vi "labview_nanonisKernel.vi"(3 "Error in (no error)":errorcluster, 4 "Input":string, 5 "Application ref in":refnum<vi>) -> (0 "Error out":errorcluster, 2 "Output":string)   [LabVIEW 2019]
uses:
  <userlib>/Nanonis Prog Interface/Scan/Grid/GridPatternGet.vi
  <userlib>/Nanonis Prog Interface/Nanonis Prog Interface.lvlib
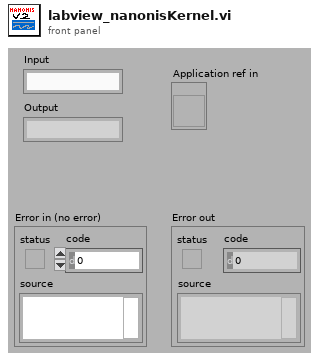
[diagram p1: front panel]
types:
  T1 = enum16{"no change", "home absolute", "home relative"}
  T2 = enum8{"Group 1", "Group 2", "Group 3", "Group 4", "Group 5", "Group 6"}
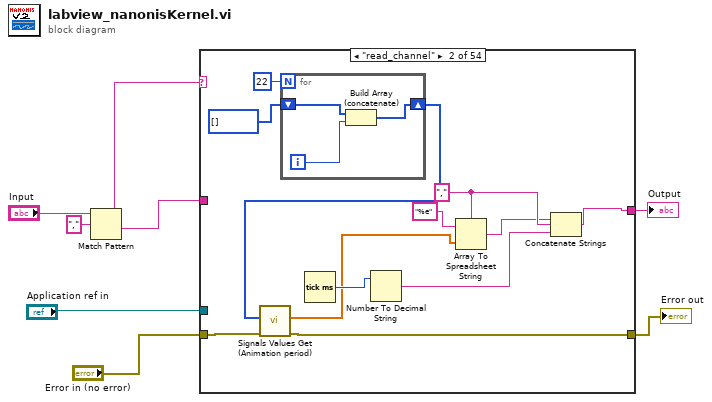
[diagram p0: block diagram]
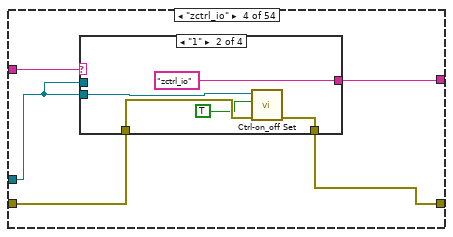
[diagram p4: hidden frame]
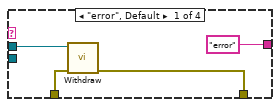
[diagram p5: hidden frame]
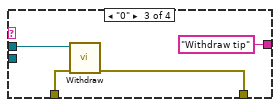
[diagram p6: hidden frame]
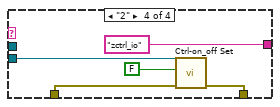
[diagram p7: hidden frame]
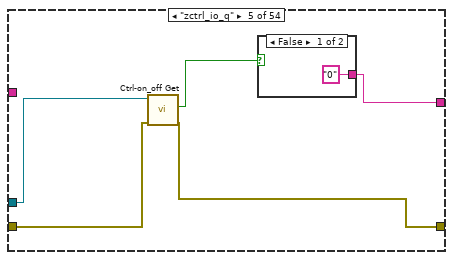
[diagram p8: hidden frame]
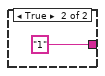
[diagram p9: hidden frame]
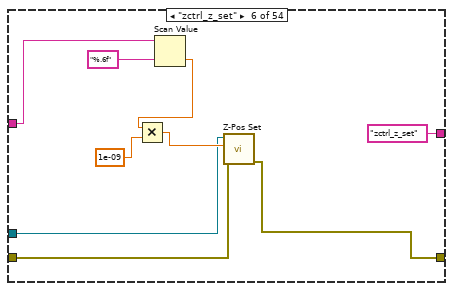
[diagram p10: hidden frame]
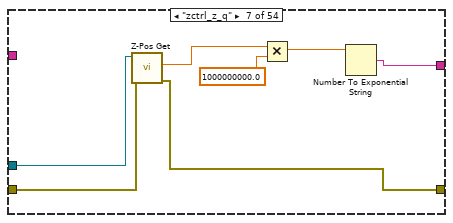
[diagram p11: hidden frame]
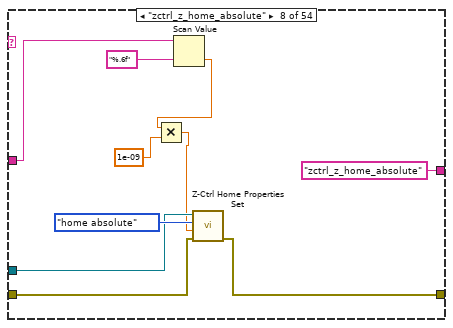
[diagram p12: hidden frame]
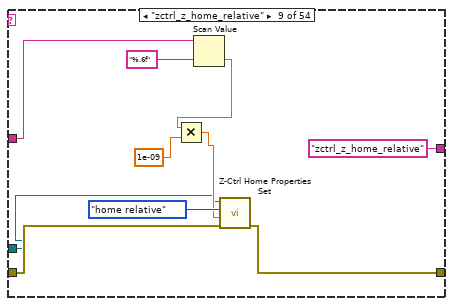
[diagram p13: hidden frame]
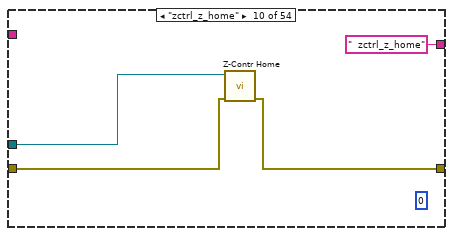
[diagram p14: hidden frame]
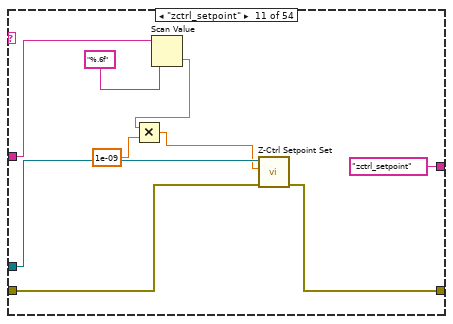
[diagram p15: hidden frame]
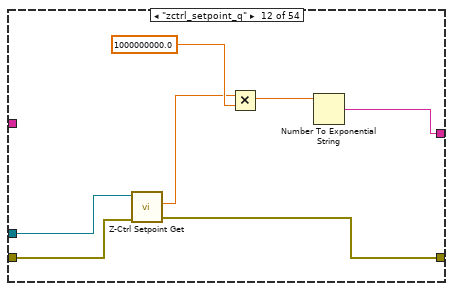
[diagram p16: hidden frame]
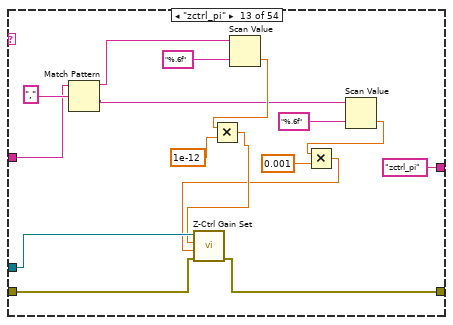
[diagram p17: hidden frame]
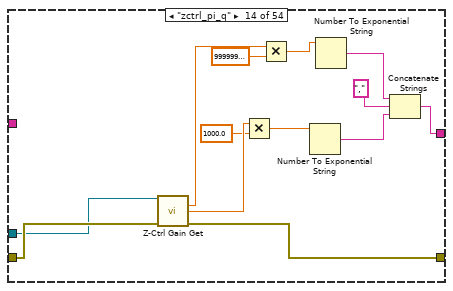
[diagram p18: hidden frame]
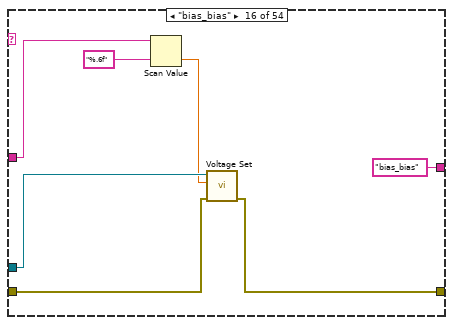
[diagram p20: hidden frame]
diagram:
  n1 = Match Pattern(string="Input", regular expression=",") -> (before substring=w5:string, after substring=w4:string)  [unwired: 1 in, 2 out]
  n2 = case shown="\"read_channel\"" w5 {
    tunnel: [w10 w12 w27 w31 w52 "zctrl_z_set" ("Input") w68 "zctrl_z_home_absolute" ("Input") "zctrl_z_home_relative" ("Input") "  zctrl_z_home" ("Input") "zctrl_setpoint" ("Input") w111 "zctrl_pi" ("Input") w130 w144 "bias_bias" ("Input") w153 "bias_pulse" ("Input") w176 w197 "bias_spec_sweep" ("Input") w216 "  bias_spec_channel" ("Input") w234 w241 w244 "walker_setting" ("Input") w264 "walker_walk" ("Input") " walker_uni_walk " ("Input") "walker_stop" ("regular expression") w344 "move_move" ("regular expression") "move_stop" ("regular expression") w370 "  move_speed" ("regular expression") w389 w397 w399 w401 w406 "lockin_setting" ("regular expression") w435 "lockin_channel" ("regular expression") w460 w479 w495 w507 w515 w530 w538 "1" ("regular expression") w552 w566] -> w8
    tunnel: w4 -> [w10 _ w27 w32 _ w65 _ w74 w84 _ w98 _ w121 _ w144 w145 _ w164 w178 _ w204 _ w230 w234 _ w244 w248 _ w270 w318 _ w344 w349 _ _ w384 _ w397 w399 w401 w402 w428 _ w451 _ w471 w496 _ w526 _ _ _ _ _]
    tunnel: "Error in (no error)" -> [w9 w22 w26 w30 w54 w60 w72 w81 w91 w97 w106 w109 w128 w142 w143 w151 w156 w171 w180 w195 w212 w221 w229 w233 w239 w243 w255 w263 w268 w325 w343 w345 w362 w366 w378 w388 w395 w396 w398 w400 w405 w434 w445 w457 w466 w486 w494 w506 _ w536 w541 w550 w556 w572]
    tunnel: "Application ref in" -> [_ _ _ w29 w55 w61 w73 w79 w85 w94 w105 w110 w127 w140 _ w148 w155 w170 w177 w194 w210 w213 w227 _ w238 _ w256 w261 w269 w326 w342 _ w361 w365 w376 w387 w393 _ _ _ w403 w432 w444 w456 w465 w487 w493 w504 w518 w537 w542 w548 w555 w573]
    tunnel: [w9 w21 w26 w28 w51 w58 w67 w80 w90 w96 w104 w108 w126 w141 w143 w150 w154 w169 w179 w196 w211 w220 w228 w233 w240 w243 w254 w262 w267 w324 w341 w345 w360 w364 w377 w380 w394 w396 w398 w400 w404 w433 w443 w455 w464 w485 w490 w505 w517 w535 w539 w549 w554 w571] -> w2
    frame "test", Default {
    }
    frame "read_channel" {
      w16 = "," ("delimiter (Tab)")
      n3 = for {
        N: 22 -> [_]
        shift-right: [w24] -> w18
        shift-left: i32[] [] -> [w25]
        i -> [w23]
        n4 = Build Array (concatenate)(w25, w23) -> (w24:i32[])
      }
      n5 = call <userlib>:"Signals Values Get (Animation period).vi"("error in (no error)"=w22, "Signals indexes (0-23)"=w18) -> ("error out"=w21:errorcluster, "Signals Values"=w11:sgl[])  [unwired: 6 in, 1 out]
      n6 = Tick Count (ms)() -> (millisecond timer value=w15:u32)
      n7 = Number To Decimal String(number=w15) -> (decimal integer string=w13:string)  [unwired: 1 in]
      n8 = Array To Spreadsheet String(delimiter (Tab)=w16, array=w11, 3:"%e" ("format string")) -> (spreadsheet string=w14:string)
      n9 = Concatenate Strings(w14, w16, w13) -> (w12:string)
    }
    frame "###z controller###" {
    }
    frame "zctrl_io" {
      n10 = case shown="\"1\"" w32 {
        tunnel: ["error" ("regular expression") "zctrl_io" ("regular expression") "Withdraw tip" ("regular expression") "zctrl_io" ("regular expression")] -> w31
        tunnel: w29 -> [w34 _ w45 _]
        tunnel: w30 -> [w35 w40 w44 w46]
        tunnel: w29 -> [_ w38 _ w48]
        tunnel: [w33 w37 w42 w49] -> w28
        frame "error", Default {
          n11 = call <userlib>:"Withdraw.vi"("Error in (no error)"=w35, "Application ref in"=w34) -> ("Error out"=w33:errorcluster)  [unwired: 8 in, 1 out]
        }
        frame "1" {
          n12 = call <userlib>:"Ctrl-on_off Set.vi"("error in (no error)"=w40, "Z Controller ON/OFF"=TRUE ("Lockin ON/OFF"), "Application ref in"=w38) -> ("error out"=w37:errorcluster)  [unwired: 7 in, 1 out]
        }
        frame "0" {
          n13 = call <userlib>:"Withdraw.vi"("Error in (no error)"=w44, "Application ref in"=w45) -> ("Error out"=w42:errorcluster)  [unwired: 8 in, 1 out]
        }
        frame "2" {
          n14 = call <userlib>:"Ctrl-on_off Set.vi"("error in (no error)"=w46, "Z Controller ON/OFF"=FALSE ("Lockin ON/OFF"), "Application ref in"=w48) -> ("error out"=w49:errorcluster)  [unwired: 7 in, 1 out]
        }
      }
    }
    frame "zctrl_io_q" {
      n15 = call <userlib>:"Ctrl-on_off Get.vi"("error in (no error)"=w54, "Application ref in"=w55) -> ("error out"=w51:errorcluster, "Z-Controller on/off status"=w53:bool)  [unwired: 7 in, 1 out]
      n16 = case shown="False" w53 {
        tunnel: ["0" "1"] -> w52
        frame False {
        }
        frame True {
        }
      }
    }
    frame "zctrl_z_set" {
      n17 = Scan Value(string=w65, format string="%.6f") -> (value=w63:dbl)  [unwired: 1 in, 1 out]
      n18 = Multiply(x=w63, y=1e-09) -> (x*y=w62:dbl)
      n19 = call <userlib>:"Z-Pos Set.vi"("error in (no error)"=w60, "Z position (m)"=w62, "Application ref in"=w61) -> ("error out"=w58:errorcluster)  [unwired: 7 in, 1 out]
    }
    frame "zctrl_z_q" {
      n20 = call <userlib>:"Z-Pos Get.vi"("error in (no error)"=w72, "Application ref in"=w73) -> ("error out"=w67:errorcluster, "Z position (m)"=w70:sgl)  [unwired: 7 in, 1 out]
      n21 = Multiply(x=w70, y=1000000000.0) -> (x*y=w69:dbl)
      n22 = Number To Exponential String(number=w69) -> (E-format string=w68:string)  [unwired: 3 in]
    }
    frame "zctrl_z_home_absolute" {
      n23 = Scan Value(string=w74, format string="%.6f") -> (value=w76:dbl)  [unwired: 1 in, 1 out]
      n24 = Multiply(x=w76, y=1e-09) -> (x*y=w75:dbl)
      n25 = call <userlib>:"Z-Ctrl Home Properties Set.vi"("error in (no error)"=w81, "Home position (m) (NaN=no change)"=w75, "Absolute/Relative Switch (no change=Default)"=T1."home absolute", "Application ref in"=w79) -> ("error out"=w80:errorcluster)  [unwired: 5 in, 1 out]
    }
    frame "zctrl_z_home_relative" {
      n26 = Scan Value(string=w84, format string="%.6f") -> (value=w87:dbl)  [unwired: 1 in, 1 out]
      n27 = Multiply(x=w87, y=1e-09) -> (x*y=w86:dbl)
      n28 = call <userlib>:"Z-Ctrl Home Properties Set.vi"("error in (no error)"=w91, "Home position (m) (NaN=no change)"=w86, "Absolute/Relative Switch (no change=Default)"=T1."home relative", "Application ref in"=w85) -> ("error out"=w90:errorcluster)  [unwired: 5 in, 1 out]
    }
    frame "zctrl_z_home" {
      (unwired) 0
      n29 = call <userlib>:"Z-Contr Home.vi"("Error in (no error)"=w97, "Application ref in"=w94) -> ("Error out"=w96:errorcluster)  [unwired: 8 in, 1 out]
    }
    frame "zctrl_setpoint" {
      n30 = Scan Value(string=w98, format string="%.6f") -> (value=w101:dbl)  [unwired: 1 in, 1 out]
      n31 = Multiply(x=w101, y=1e-09) -> (x*y=w100:dbl)
      n32 = call <userlib>:"Z-Ctrl Setpoint Set.vi"("error in (no error)"=w106, "Z Controller setpoint"=w100, "Application ref in"=w105) -> ("error out"=w104:errorcluster)  [unwired: 7 in, 1 out]
    }
    frame "zctrl_setpoint_q" {
      n33 = call <userlib>:"Z-Ctrl Setpoint Get.vi"("error in (no error)"=w109, "Application ref in"=w110) -> ("error out"=w108:errorcluster, "Z Controller setpoint"=w107:sgl)  [unwired: 6 in, 1 out]
      n34 = Multiply(x=w107, y=1000000000.0) -> (x*y=w112:dbl)
      n35 = Number To Exponential String(number=w112) -> (E-format string=w111:string)  [unwired: 3 in]
    }
    frame "zctrl_pi" {
      n36 = Match Pattern(string=w121, regular expression=",") -> (before substring=w120:string, after substring=w117:string)  [unwired: 1 in, 2 out]
      n37 = Scan Value(string=w120, format string="%.6f") -> (value=w123:dbl)  [unwired: 1 in, 1 out]
      n38 = Multiply(x=w123, y=1e-12) -> (x*y=w119:dbl)
      n39 = Scan Value(string=w117, format string="%.6f") -> (value=w116:dbl)  [unwired: 1 in, 1 out]
      n40 = Multiply(x=w116, y=0.001) -> (x*y=w115:dbl)
      n41 = call <userlib>:"Z-Ctrl Gain Set.vi"("error in (no error)"=w128, "Time constant (s)"=w115, "P-gain"=w119, "Application ref in"=w127) -> ("error out"=w126:errorcluster)  [unwired: 5 in, 1 out]
    }
    frame "zctrl_pi_q" {
      n42 = call <userlib>:"Z-Ctrl Gain Get.vi"("Application ref in"=w140, "error in (no error)"=w142) -> ("P-gain"=w137:sgl, "Time constant (s)"=w136:sgl, "error out"=w141:errorcluster)  [unwired: 9 in, 2 out]
      n43 = Multiply(x=w136, y=sgl 1000.0) -> (x*y=w138:sgl)
      n44 = Multiply(x=w137, y=sgl 1000000000000.0) -> (x*y=w139:sgl)
      n45 = Number To Exponential String(number=w138) -> (E-format string=w131:string)  [unwired: 3 in]
      n46 = Number To Exponential String(number=w139) -> (E-format string=w132:string)  [unwired: 3 in]
      n47 = Concatenate Strings(w132, "," ("string"), w131) -> (w130:string)
    }
    frame "###Bias/Bias Spectrum###" {
    }
    frame "bias_bias" {
      n48 = Scan Value(string=w145, format string="%.6f") -> (value=w147:dbl)  [unwired: 1 in, 1 out]
      n49 = call <userlib>:"Voltage Set.vi"("Error in (no error)"=w151, "Bias (V)"=w147, "Application ref in"=w148) -> ("Error out"=w150:errorcluster)  [unwired: 7 in, 1 out]
    }
    frame "bias_bias_q" {
      n50 = call <userlib>:"Voltage Get.vi"("error in (no error)"=w156, "Application ref in"=w155) -> ("error out"=w154:errorcluster, "Bias (V)"=w152:sgl)  [unwired: 7 in, 1 out]
      n51 = Number To Exponential String(number=w152) -> (E-format string=w153:string)  [unwired: 3 in]
    }
    frame "bias_pulse" {
      w161 = "," ("regular expression")
      n52 = Match Pattern(string=w164, regular expression=w161) -> (before substring=w166:string, after substring=w159:string)  [unwired: 1 in, 2 out]
      n53 = Match Pattern(string=w159, regular expression=w161) -> (before substring=w160:string, after substring=w158:string)  [unwired: 1 in, 2 out]
      n54 = Scan Value(string=w166, format string="%.6f") -> (value=w163:dbl)  [unwired: 1 in, 1 out]
      n55 = case shown="\"0\"" w158 {
        tunnel: [enum16{"no change", "hold", "don't hold"}."no change" ("Z-Controller (no change)") enum16{"no change", "hold", "don't hold"}."hold" ("Z-Controller (no change)") enum16{"no change", "hold", "don't hold"}."don't hold" ("Z-Controller (no change)")] -> w157
        frame Default {
        }
        frame "1" {
        }
        frame "0" {
        }
      }
      n56 = Scan Value(string=w160, format string="%.6f") -> (value=w162:dbl)  [unwired: 1 in, 1 out]
      n57 = call <userlib>:"Bias Pulse.vi"("Application ref in"=w170, "Pulse bias (V) (1)"=w163, "Pulse width (s) (100m)"=w162, "Z-Controller (no change)"=w157, "Error in (no error)"=w171, "Pulse abs/rel (no change)"=enum16{"no change", "relative", "absolute"}."absolute") -> ("Error out"=w169:errorcluster)  [unwired: 8 in, 1 out]
    }
    frame "bias_spec_io" {
      n58 = case shown="\"1\"" w178 {
        tunnel: ["Error!" ("regular expression") w185 "STS stop" ("regular expression")] -> w176
        tunnel: w180 -> [w181 w189 w192]
        tunnel: w177 -> [_ w190 _]
        tunnel: [w181 w188 w191] -> w179
        frame "error", Default {
        }
        frame "1" {
          n59 = call <userlib>:"BiasSpectroscopy Start.vi"("Application ref in"=w190, "Get data (F)"=TRUE, "Error in (no error)"=w189) -> ("Data"=w184:sgl[][], "Error out"=w188:errorcluster)  [unwired: 8 in, 3 out]
          n60 = Array To Spreadsheet String(delimiter (Tab)=",", array=w184, 3:"%e" ("format string")) -> (spreadsheet string=w185:string)
        }
        frame "0" {
          n61 = call <userlib>:"BiasSpectroscopy Stop.vi"("Error in (no error)"=w192) -> ("Error out"=w191:errorcluster)  [unwired: 13 in, 1 out]
        }
      }
    }
    frame "bias_spec_q" {
      n62 = call <userlib>:"BiasSpectroscopy Status Get.vi"("Error in (no error)"=w195, "Application ref in"=w194) -> ("Error out"=w196:errorcluster, "Running?"=w198:bool)  [unwired: 5 in, 1 out]
      n63 = case shown="True" w198 {
        tunnel: ["0" "1"] -> w197
        frame False {
        }
        frame True {
        }
      }
    }
    frame "bias_spec_sweep" {
      n64 = Match Pattern(string=w204, regular expression=",") -> (before substring=w207:string, after substring=w205:string)  [unwired: 1 in, 2 out]
      n65 = Scan Value(string=w207, format string="%.6f") -> (value=w203:dbl)  [unwired: 1 in, 1 out]
      n66 = Scan Value(string=w205, format string="%.6f") -> (value=w202:dbl)  [unwired: 1 in, 1 out]
      n67 = call <userlib>:"BiasSpectroscopy SetLimits.vi"("Error in (no error)"=w212, "End value (V)"=w202, "Start value (V)"=w203, "Application ref in"=w210) -> ("Error out"=w211:errorcluster)  [unwired: 4 in, 1 out]
    }
    frame "bias_spec_sweep_q" {
      n68 = call <userlib>:"BiasSpectroscopy GetLimits.vi"("Error in (no error)"=w221, "Application ref in"=w213) -> ("Error out"=w220:errorcluster, "End value (V)"=w215:sgl, "Start value (V)"=w214:sgl)  [unwired: 4 in, 1 out]
      n69 = Number To Exponential String(number=w215) -> (E-format string=w217:string)  [unwired: 3 in]
      n70 = Number To Exponential String(number=w214) -> (E-format string=w218:string)  [unwired: 3 in]
      n71 = Concatenate Strings(w218, "," ("string"), w217) -> (w216:string)
    }
    frame "bias_spec_channel" {
      n72 = Spreadsheet String To Array(delimiter (Tab)=",", format string="", spreadsheet string=w230) -> (array=w225:dbl[][])  [unwired: 1 in]
      n73 = Array Size(array=w225) -> (size(s)=w226:i32[])
      n74 = Array Max & Min(array=w226) -> (max value=w224:i32)  [unwired: 3 out]
      n75 = Reshape Array(w225, w224) -> (w223:dbl[])
      n76 = call <userlib>:"BiasSpectroscopy Channels Set.vi"("Error in (no error)"=w229, "Channels"=w223, "Application ref in"=w227) -> ("Error out"=w228:errorcluster)  [unwired: 7 in, 1 out]
    }
    frame "###Current###" {
    }
    frame "current" {
      n77 = call <userlib>:"Current Get.vi"("Error in (no error)"=w239, "Application ref in"=w238) -> ("Error out"=w240:errorcluster, "Current (A)"=w237:sgl)  [unwired: 5 in, 1 out]
      n78 = Multiply(x=sgl 1000000000.0, y=w237) -> (x*y=w236:sgl)
      n79 = Format Value(format string="%e", value (0)=w236) -> (output string=w241:string)  [unwired: 1 in]
    }
    frame "###Walker###" {
    }
    frame "walker_setting" {
      n80 = Match Pattern(string=w248, regular expression=",") -> (before substring=w251:string, after substring=w249:string)  [unwired: 1 in, 2 out]
      n81 = Scan Value(string=w251, format string="%.6f") -> (value=w247:dbl)  [unwired: 1 in, 1 out]
      n82 = Scan Value(string=w249, format string="%.6f") -> (value=w246:dbl)  [unwired: 1 in, 1 out]
      n83 = call <userlib>:"Motor Frequency Amplitude Set.vi"("Error in (no error)"=w255, "Amplitude (V) (NaN=no change)"=w247, "Frequency (Hz) (NaN=no change)"=w246, "Application ref in"=w256) -> ("Error out"=w254:errorcluster)  [unwired: 6 in, 1 out]
    }
    frame "walker_setting_q" {
      n84 = call <userlib>:"Motor Frequency Amplitude Get.vi"("Error in (no error)"=w263, "Application ref in"=w261) -> ("Error out"=w262:errorcluster, "Amplitude (V)"=w260:sgl, "Frequency (Hz)"=w258:sgl)  [unwired: 6 in, 1 out]
      n85 = Number To Decimal String(number=w258) -> (decimal integer string=w257:string)  [unwired: 1 in]
      n86 = Number To Decimal String(number=w260) -> (decimal integer string=w259:string)  [unwired: 1 in]
      n87 = Concatenate Strings(w259, "," ("string"), w257) -> (w264:string)
    }
    frame "walker_walk" {
      n88 = Match Pattern(string=w270, regular expression=",") -> (before substring=w275:string, after substring=w273:string)  [unwired: 1 in, 2 out]
      n89 = Scan Value(string=w275, format string="%d") -> (value=w271:dbl)  [unwired: 1 in, 1 out]
      n90 = Scan Value(string=w273, format string="%d") -> (value=w272:dbl)  [unwired: 1 in, 1 out]
      n91 = case shown="2" w271 {
        tunnel: w269 -> [_ w284 w290 w296 w302 w308 w310]
        tunnel: w268 -> [w278 w283 w289 w295 w301 w307 w313]
        tunnel: [w278 w282 w288 w294 w300 w306 w312] -> w267
        tunnel: w272 -> [_ w280 w286 w292 w298 w304 w311]
        frame 0, Default {
        }
        frame 1 {
          n92 = call <userlib>:"Motor Start Move.vi"("Group"=T2."Group 4", "Error in (no error)"=w283, "Number of steps"=w280, "Direction"=enum16{"X +", "X -", "Y +", "Y -", "Z +", "Z -"}."X +", "Application ref in"=w284) -> ("Error out"=w282:errorcluster)  [unwired: 4 in, 1 out]
        }
        frame 2 {
          n93 = call <userlib>:"Motor Start Move.vi"("Group"=T2."Group 4", "Error in (no error)"=w289, "Number of steps"=w286, "Direction"=enum16{"X +", "X -", "Y +", "Y -", "Z +", "Z -"}."X -", "Application ref in"=w290) -> ("Error out"=w288:errorcluster)  [unwired: 4 in, 1 out]
        }
        frame 3 {
          n94 = call <userlib>:"Motor Start Move.vi"("Group"=T2."Group 4", "Error in (no error)"=w295, "Number of steps"=w292, "Direction"=enum16{"X +", "X -", "Y +", "Y -", "Z +", "Z -"}."Y +", "Application ref in"=w296) -> ("Error out"=w294:errorcluster)  [unwired: 4 in, 1 out]
        }
        frame 4 {
          n95 = call <userlib>:"Motor Start Move.vi"("Group"=T2."Group 4", "Error in (no error)"=w301, "Number of steps"=w298, "Direction"=enum16{"X +", "X -", "Y +", "Y -", "Z +", "Z -"}."Y -", "Application ref in"=w302) -> ("Error out"=w300:errorcluster)  [unwired: 4 in, 1 out]
        }
        frame 5 {
          n96 = call <userlib>:"Motor Start Move.vi"("Group"=T2."Group 4", "Error in (no error)"=w307, "Number of steps"=w304, "Direction"=enum16{"X +", "X -", "Y +", "Y -", "Z +", "Z -"}."Z +", "Application ref in"=w308) -> ("Error out"=w306:errorcluster)  [unwired: 4 in, 1 out]
        }
        frame 6 {
          n97 = call <userlib>:"Motor Start Move.vi"("Group"=T2."Group 4", "Error in (no error)"=w313, "Number of steps"=w311, "Direction"=enum16{"X +", "X -", "Y +", "Y -", "Z +", "Z -"}."Z -", "Application ref in"=w310) -> ("Error out"=w312:errorcluster)  [unwired: 4 in, 1 out]
        }
      }
    }
    frame "walker_uni_walk" {
      n98 = Match Pattern(string=w318, regular expression=",") -> (before substring=w321:string, after substring=w319:string)  [unwired: 1 in, 2 out]
      n99 = Scan Value(string=w321, format string="%d") -> (value=w316:dbl)  [unwired: 1 in, 1 out]
      n100 = Scan Value(string=w319, format string="%d") -> (value=w317:dbl)  [unwired: 1 in, 1 out]
      n101 = case shown="0, Default" w316 {
        tunnel: w326 -> [_ w333 w335]
        tunnel: w325 -> [w327 w332 w338]
        tunnel: [w327 w331 w337] -> w324
        tunnel: w317 -> [_ w329 w336]
        frame 0, Default {
        }
        frame 5 {
          n102 = call <userlib>:"Motor Start Move.vi"("Group"=T2."Group 5", "Error in (no error)"=w332, "Number of steps"=w329, "Direction"=enum16{"X +", "X -", "Y +", "Y -", "Z +", "Z -"}."Z +", "Application ref in"=w333) -> ("Error out"=w331:errorcluster)  [unwired: 4 in, 1 out]
        }
        frame 6 {
          n103 = call <userlib>:"Motor Start Move.vi"("Group"=T2."Group 5", "Error in (no error)"=w338, "Number of steps"=w336, "Direction"=enum16{"X +", "X -", "Y +", "Y -", "Z +", "Z -"}."Z -", "Application ref in"=w335) -> ("Error out"=w337:errorcluster)  [unwired: 4 in, 1 out]
        }
      }
    }
    frame "walker_stop" {
      n104 = call <userlib>:"Motor Stop Move.vi"("Error in (no error)"=w343, "Application ref in"=w342) -> ("Error out"=w341:errorcluster)  [unwired: 8 in, 1 out]
    }
    frame "###Move/Drift/Tilt###" {
    }
    frame "move_move" {
      n105 = Match Pattern(string=w349, regular expression=",") -> (before substring=w354:string, after substring=w352:string)  [unwired: 1 in, 2 out]
      n106 = Scan Value(string=w354, format string="%.6f") -> (value=w356:dbl)  [unwired: 1 in, 1 out]
      n107 = Multiply(x=w356, y=1e-09) -> (x*y=w348:dbl)
      n108 = Scan Value(string=w352, format string="%.6f") -> (value=w350:dbl)  [unwired: 1 in, 1 out]
      n109 = Multiply(x=w350, y=1e-09) -> (x*y=w347:dbl)
      n110 = call <userlib>:"XY-Pos Set - Fast.vi"("Wait end-of-motion (T=True)"=FALSE, "error in (no error)"=w362, "Y (m)"=w347, "X (m)"=w348, "Application ref in"=w361) -> ("error out"=w360:errorcluster)  [unwired: 4 in, 1 out]
    }
    frame "move_stop" {
      n111 = call <userlib>:"FolMe Stop Movement.vi"("error in (no error)"=w366, "Application ref in"=w365) -> ("error out"=w364:errorcluster)  [unwired: 6 in, 1 out]
    }
    frame "move_q" {
      w367 = sgl 1000000000.0 ("y")
      n112 = call <userlib>:"XY-Pos Get.vi"("error in (no error)"=w378, "Application ref in"=w376) -> ("error out"=w377:errorcluster, "Y (m)"=w368:sgl, "X (m)"=w369:sgl)  [unwired: 5 in, 1 out]
      n113 = Multiply(x=w368, y=w367) -> (x*y=w374:sgl)
      n114 = Multiply(x=w369, y=w367) -> (x*y=w375:sgl)
      n115 = Number To Exponential String(number=w374) -> (E-format string=w371:string)  [unwired: 3 in]
      n116 = Number To Exponential String(number=w375) -> (E-format string=w372:string)  [unwired: 3 in]
      n117 = Concatenate Strings(w372, "," ("string"), w371) -> (w370:string)
    }
    frame "move_speed" {
      n118 = Scan Value(string=w384, format string="%.6f") -> (value=w382:dbl)  [unwired: 1 in, 1 out]
      n119 = Multiply(x=w382, y=1e-09) -> (x*y=w379:dbl)
      n120 = call <userlib>:"FolMe Speed Set.vi"("error in (no error)"=w388, "Speed Setting (Custom)"=enum32{"Scan speed", "Custom speed"}."Custom speed", "Speed (m/s)"=w379, "Application ref in"=w387) -> ("error out"=w380:errorcluster)  [unwired: 4 in, 1 out]
    }
    frame "move_speed_q" {
      n121 = call <userlib>:"FolMe Speed Get.vi"("error in (no error)"=w395, "Application ref in"=w393) -> ("error out"=w394:errorcluster, "Speed (m/s)"=w390:sgl)  [unwired: 4 in, 2 out]
      n122 = Multiply(x=w390, y=sgl 1000000000.0) -> (x*y=w392:sgl)
      n123 = Number To Exponential String(number=w392) -> (E-format string=w389:string)  [unwired: 3 in]
    }
    frame "###Scan###" {
    }
    frame "###Grid###" {
    }
    frame "###LockIn###" {
    }
    frame "lockin_io" {
      n124 = case shown="\"error\", Default" w402 {
        tunnel: ["error" ("regular expression") "lockin off" ("regular expression") "lockin on" ("regular expression")] -> w406
        tunnel: w405 -> [w407 w412 w417]
        tunnel: w403 -> [_ w410 w415]
        tunnel: [w407 w411 w416] -> w404
        frame "error", Default {
        }
        frame "0" {
          n125 = call <userlib>:"Lockin on_off Set.vi"("Error in (no error)"=w412, "Lockin ON/OFF"=FALSE, "Application ref in"=w410) -> ("Error out"=w411:errorcluster)  [unwired: 7 in, 1 out]
        }
        frame "1" {
          n126 = call <userlib>:"Lockin on_off Set.vi"("Error in (no error)"=w417, "Lockin ON/OFF"=TRUE, "Application ref in"=w415) -> ("Error out"=w416:errorcluster)  [unwired: 7 in, 1 out]
        }
      }
    }
    frame "lockin_setting" {
      w426 = "," ("regular expression")
      n127 = Match Pattern(string=w428, regular expression=w426) -> (before substring=w431:string, after substring=w427:string)  [unwired: 1 in, 2 out]
      n128 = Match Pattern(string=w427, regular expression=w426) -> (before substring=w425:string, after substring=w423:string)  [unwired: 1 in, 2 out]
      n129 = Scan Value(string=w431, format string="%.6f") -> (value=w422:dbl)  [unwired: 1 in, 1 out]
      n130 = Scan Value(string=w425, format string="%.6f") -> (value=w421:dbl)  [unwired: 1 in, 1 out]
      n131 = Scan Value(string=w423, format string="%.6f") -> (value=w420:dbl)  [unwired: 1 in, 1 out]
      n132 = call <userlib>:"Lockin Modulation param Set.vi"("Application ref in"=w432, "Amplitude (mod. signal unit) (NaN = no change)"=w422, "Frequency (Hz) (NaN = no change)"=w421, "Ref Phase (deg) (NaN = no change)"=w420, "Error in (no error)"=w434) -> ("Error out"=w433:errorcluster)  [unwired: 9 in, 1 out]
    }
    frame "lockin_setting_q" {
      w440 = "," ("string")
      n133 = call <userlib>:"Lockin Modulation param Get.vi"("Application ref in"=w444, "Error in (no error)"=w445) -> ("Amplitude (mod. signal unit)"=w438:sgl, "Frequency (Hz)"=w437:sgl, "Ref phase (deg)"=w436:sgl, "Error out"=w443:errorcluster)  [unwired: 9 in, 1 out]
      n134 = Number To Exponential String(number=w436) -> (E-format string=w439:string)  [unwired: 3 in]
      n135 = Number To Exponential String(number=w437) -> (E-format string=w441:string)  [unwired: 3 in]
      n136 = Number To Exponential String(number=w438) -> (E-format string=w442:string)  [unwired: 3 in]
      n137 = Concatenate Strings(w442, w440, w441, w440, w439) -> (w435:string)
    }
    frame "lockin_channel" {
      n138 = Match Pattern(string=w451, regular expression=",") -> (before substring=w450:string, after substring=w449:string)  [unwired: 1 in, 2 out]
      n139 = Scan Value(string=w450, format string="%d") -> (value=w448:dbl)  [unwired: 1 in, 1 out]
      n140 = Scan Value(string=w449, format string="%d") -> (value=w447:dbl)  [unwired: 1 in, 1 out]
      n141 = call <userlib>:"Lockin MoDem Signal Set.vi"("Error in (no error)"=w457, "Demod. index"=w447, "Mod. index"=w448, "Application ref in"=w456) -> ("Error out"=w455:errorcluster)  [unwired: 6 in, 1 out]
    }
    frame "lockin_channel_q" {
      n142 = call <userlib>:"Lockin MoDem Signal Get.vi"("Error in (no error)"=w466, "Application ref in"=w465) -> ("Error out"=w464:errorcluster, "Demod. signal index"=w458:i8, "Mod. signal index"=w459:i8)  [unwired: 6 in, 1 out]
      n143 = Number To Exponential String(number=w458) -> (E-format string=w461:string)  [unwired: 3 in]
      n144 = Number To Exponential String(number=w459) -> (E-format string=w462:string)  [unwired: 3 in]
      n145 = Concatenate Strings(w462, "," ("string"), w461) -> (w460:string)
    }
    frame "APP" {
      w467 = "," ("regular expression")
      # "100ms"
      n146 = Match Pattern(string=w471, regular expression=w467) -> (before substring=w477:string, after substring=w478:string)  [unwired: 1 in, 2 out]
      n147 = Match Pattern(string=w478, regular expression=w467) -> (before substring=w476:string, after substring=w468:string)  [unwired: 1 in, 2 out]
      n148 = Match Pattern(string=w468, regular expression=w467) -> (before substring=w469:string)  [unwired: 1 in, 3 out]
      n149 = Decimal String To Number(string=w469) -> (number=w470:i32)  [unwired: 2 in, 1 out]
      n150 = Decimal String To Number(string=w476) -> (number=w474:i32)  [unwired: 2 in, 1 out]
      n151 = Multiply(x=w474, y=1000) -> (x*y=w472:i32)
      n152 = Decimal String To Number(string=w477) -> (number=w475:i32)  [unwired: 2 in, 1 out]
      n153 = call "Nanonis_autoAPP.vi"("Application reference"=w487, "steps"=w475, "Number of pulses"=w470, "Wait for motor (ms)"=w472, "Error in (no error)"=w486) -> ("Surface reached"=w484:bool, "Total steps"=w480:u32, "error out"=w485:errorcluster)  [unwired: 1 in]
      n154 = case shown="False" w484 {
        tunnel: ["0" ("regular expression") "1" ("regular expression")] -> w483
        frame False {
        }
        frame True {
        }
      }
      n155 = Number To Decimal String(number=w480) -> (decimal integer string=w481:string)  [unwired: 1 in]
      n156 = Concatenate Strings(w483, "," ("string"), w481) -> (w479:string)
    }
    frame "SCAN_IO" {
      (unwired) 0
      n157 = case shown="\"start\"" w496 {
        tunnel: ["Error!" ("regular expression") "Scan start" ("regular expression") "Scan stop" ("regular expression")] -> w495
        tunnel: [enum16{"Start", "Stop", "Pause", "Resume"}."Pause" ("Scan action (Start)") enum16{"Start", "Stop", "Pause", "Resume"}."Start" ("Scan action (Start)") enum16{"Start", "Stop", "Pause", "Resume"}."Stop" ("Scan action (Start)")] -> w492
        frame "error", Default {
        }
        frame "start" {
        }
        frame "stop" {
          (unwired) FALSE ("Lockin ON/OFF")
        }
      }
      n158 = call <userlib>:"Scan Action.vi"("error in (no error)"=w494, "Direction: up/down (T=up)"=TRUE, "Scan action (Start)"=w492, "Application ref in"=w493) -> ("error out"=w490:errorcluster)  [unwired: 5 in, 1 out]
    }
    frame "SCAN_STAT" {
      (unwired) 0
      n159 = call <userlib>:"Scan Status Get.vi"("error in (no error)"=w506, "Application ref in"=w504) -> ("error out"=w505:errorcluster, "Scanning?"=w503:bool)  [unwired: 6 in, 1 out]
      n160 = case shown="False" w503 {
        tunnel: ["0" "1"] -> w507
        frame False {
        }
        frame True {
        }
      }
    }
    frame "SCAN_FRAME" {
      (unwired) 0
      w521 = "," ("regular expression")
      # "size"
      # "Y"
      # "X"
      n161 = Match Pattern(string=w526, regular expression=w521) -> (before substring=w514:string, after substring=w527:string)  [unwired: 1 in, 2 out]
      n162 = Match Pattern(string=w527, regular expression=w521) -> (before substring=w512:string, after substring=w522:string)  [unwired: 1 in, 2 out]
      n163 = Match Pattern(string=w522, regular expression=w521) -> (before substring=w510:string)  [unwired: 1 in, 3 out]
      n164 = Fract/Exp String To Number(string=w514) -> (number=w525:dbl)  [unwired: 3 in, 1 out]
      n165 = Fract/Exp String To Number(string=w512) -> (number=w524:dbl)  [unwired: 3 in, 1 out]
      n166 = Fract/Exp String To Number(string=w510) -> (number=w520:dbl)  [unwired: 3 in, 1 out]
      n167 = Bundle(w520, w520) -> (w519:cluster{dbl, dbl})  [unwired: 1 in]
      n168 = Bundle(w525, w524) -> (w523:cluster{dbl, dbl})  [unwired: 1 in]
      n169 = call <userlib>:"ScanFrame Set.vi"("Application ref in"=w518, "Center coordinates (m)"=w523, "Size (m)"=w519) -> ("error out"=w517:errorcluster)  [unwired: 11 in, 1 out]
      n170 = Concatenate Strings("Frame set: X= " ("string"), w514, ", Y= " ("string"), w512, ", size= " ("string"), w510) -> (w515:string)
    }
    frame "SCAN_location" {
      (unwired) 0
      n171 = call <userlib>:"ScanFrame Get.vi"("Application ref in"=w537, "error in (no error)"=w536) -> ("Center coordinates (m)"=w534:cluster{"Xc":sgl, "Yc":sgl}, "error out"=w535:errorcluster)  [unwired: 9 in, 3 out]
      n172 = Unbundle(w534) -> ("Xc"=w532:sgl, "Yc"=w531:sgl)
      n173 = Number To Exponential String(number=w532) -> (E-format string=w533:string)  [unwired: 3 in]
      n174 = Number To Exponential String(number=w531) -> (E-format string=w529:string)  [unwired: 3 in]
      n175 = Concatenate Strings(w533, "," ("string"), w529) -> (w530:string)
    }
    frame "SCAN_size" {
      n176 = call <userlib>:"ScanFrame Get.vi"("Application ref in"=w542, "error in (no error)"=w541) -> ("Size (m)"=w540:cluster{"Width":sgl, "Height":sgl}, "error out"=w539:errorcluster)  [unwired: 9 in, 3 out]
      n177 = Unbundle(w540) -> ("Width"=w546:sgl, "Height"=w545:sgl)
      n178 = Number To Exponential String(number=w546) -> (E-format string=w547:string)  [unwired: 3 in]
      n179 = Number To Exponential String(number=w545) -> (E-format string=w544:string)  [unwired: 3 in]
      n180 = Concatenate Strings(w547, "," ("string"), w544) -> (w538:string)
    }
    frame "GRD_IO" {
      (unwired) 1
      n181 = call <userlib>:"Start Grid Experiment.vi"("Application ref in"=w548, "error in (no error)"=w550) -> ("error out"=w549:errorcluster)  [unwired: 16 in, 1 out]
    }
    frame "GRD_STAT" {
      (unwired) 0
      n182 = call <userlib>:"Grid Experiment Status Get.vi"("error in (no error)"=w556, "Application ref in"=w555) -> ("error out"=w554:errorcluster, "Running?"=w553:bool)  [unwired: 7 in, 1 out]
      n183 = case shown="False" w553 {
        tunnel: ["0" "1"] -> w552
        frame False {
        }
        frame True {
        }
      }
    }
    frame "GRD_pattn" {
      w561 = "," ("string")
      (unwired) 0
      n184 = call-poly <userlib>:"Grid Pattern Get.vi"("Application ref in"=w573, "error in (no error)"=w572) -> ("Height (m)"=w562:sgl, "Width (m)"=w563:sgl, "Center Xc (m)"=w565:sgl, "Center Yc (m)"=w564:sgl, "Angle (°)"=w559:sgl, "error out"=w571:errorcluster)  [unwired: 9 in, 3 out]
      n185 = Number To Exponential String(number=w562) -> (E-format string=w567:string)  [unwired: 3 in]
      n186 = Number To Exponential String(number=w565) -> (E-format string=w570:string)  [unwired: 3 in]
      n187 = Number To Exponential String(number=w564) -> (E-format string=w569:string)  [unwired: 3 in]
      n188 = Number To Exponential String(number=w563) -> (E-format string=w568:string)  [unwired: 3 in]
      n189 = Number To Exponential String(number=w559) -> (E-format string=w560:string)  [unwired: 3 in]
      n190 = Concatenate Strings(w570, w561, w569, w561, w568, w561, w567, w561, w560) -> (w566:string)
    }
  }
  "Output" <- w8
  "Error out" <- w2
